vi "Queues - Get.vi"(8 "error in":errorcluster) -> (0 "error out":errorcluster, 3 "Queues Out":T1)   [LabVIEW 2024, in "ECU InterComm.lvlib"]
uses:
  ECU InterComm.lvlib
  General Actions.ctl
  QMH Item.ctl
  Process Queues.ctl
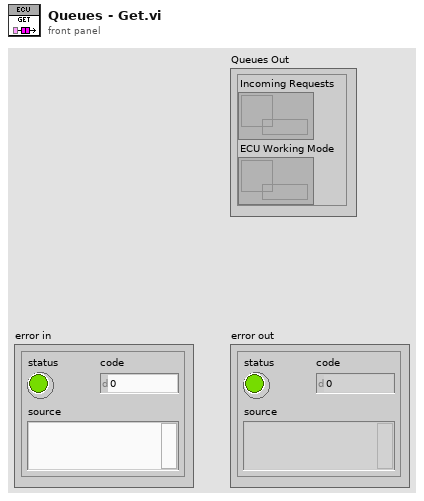
[diagram p1: front panel]
types:
  T1 = typedef "ECU InterComm.lvlib/Process Queues.ctl" = cluster{"Incoming Requests":refnum<queue>, "ECU Working Mode":refnum<queue>}
  T2 = typedef "ECU InterComm.lvlib/General Actions.ctl" = enum16{"Create", "Get", "Destroy"}
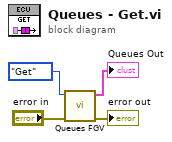
[diagram p0: block diagram]
diagram:
  n1 = call "Queues FGV.vi"("error in"="error in", "Action"=General_Actions."Get") -> ("error out"=→"error out":errorcluster, "Queues Out"=→"Queues Out":T1)  [unwired: 8 in]
